vi "Instrument Handle Diaog.vi"(8 "error in":errorcluster, 10 "Devices in":string[](array[string]), 11 "Config in":refnum<class "Config.lvclass">) -> (0 "error out":errorcluster, 1 "Cancelled?":bool, 3 "Config out":refnum<class "Config.lvclass">)   [LabVIEW 2023, in "Config.lvlib" / "Config.lvclass"]
uses:
  Config.lvclass
  Config.lvclass/Config.ctl
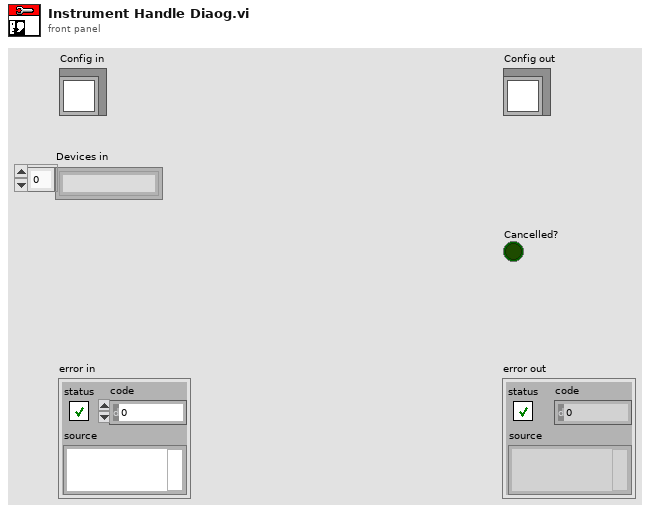
[diagram p1: front panel]
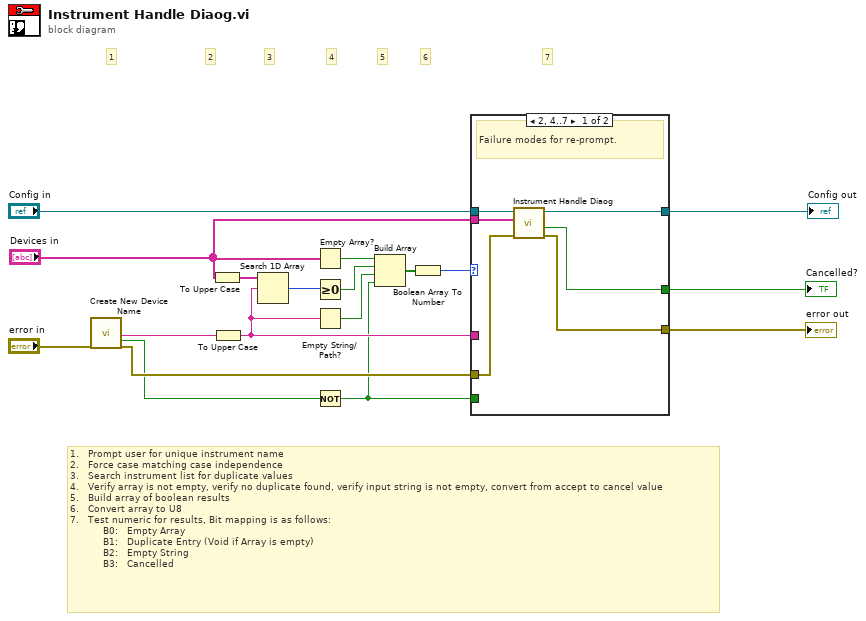
[diagram p0: block diagram]
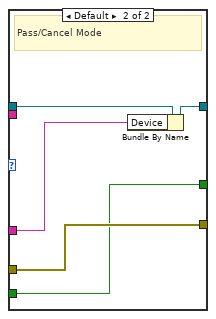
[diagram p2: hidden frame]
diagram:
  # "1.   Prompt user for unique instrument name\n2.   Force case matching case independence\n3.   Search instrument list for duplicate values\n4.   Verify array is not empty, verify no duplicate found, verify input string is not empty, convert from accept to cancel value\n5.   Build array of boolean results\n6.   Convert array to U8\n7.   Test numeric for results, Bit mapping is as follows:\n           B0:   Empty Array \n           B1:   Duplicate Entry (Void if Array is empty)\n           B2:   Empty String\n           B3:   Cancelled"
  # "7"
  # "6"
  # "5"
  # "4"
  # "3"
  # "2"
  # "1"
  n1 = call "Create New Device Name"("error in (no error)"="error in") -> ("Instrument Name"=w17:string, "Accept"=w5:bool, "error out"=w10:errorcluster)  [unwired: 16 in]
  n2 = To Upper Case(1:"Devices in") -> (0:w16:string[])
  n3 = To Upper Case(1:w17) -> (0:w9:string)
  n4 = Search 1D Array(1D array=w16, element=w9) -> (index of element=w15:i32)  [unwired: 1 in]
  n5 = Empty Array?(array="Devices in") -> (empty?=w7:bool)
  n6 = Greater Or Equal To 0?(x=w15) -> (x >= 0?=w3:bool)
  n7 = Empty String/Path?(string/path=w9) -> (empty?=w6:bool)
  n8 = Not(x=w5) -> (.not. x?=w2:bool)
  n9 = Build Array(w7, w3, w6, w2) -> (w4:bool[])
  n10 = Boolean Array To Number(Boolean array=w4) -> (number=w1:u32)
  n11 = case shown="2, 4..7" w1 {
    tunnel: w9 -> [_ w25]
    tunnel: [w21 w27] -> w12
    tunnel: "Config in" -> [w24 w29]
    tunnel: [w23 w26] -> w13
    tunnel: "Devices in" -> [w22 _]
    tunnel: [w20 w28] -> w11
    tunnel: w10 -> [w19 w28]
    tunnel: w2 -> [_ w27]
    frame 2, 4..7 {
      # "Failure modes for re-prompt."
      n12 = call "Instrument Handle Diaog.vi"("error in"=w19, "Devices in"=w22, "Config in"=w24) -> ("error out"=w20:errorcluster, "Cancelled?"=w21:bool, "Config out"=w23:refnum<class "Config.lvclass">)  [unwired: 6 in]
    }
    frame Default {
      # "Pass/Cancel Mode"
      n13 = Bundle By Name(cluster=w29, "Device"=w25) -> (w26:refnum<class "Config.lvclass">)
    }
  }
  "error out" <- w11
  "Config out" <- w13
  "Cancelled?" <- w12
